vi "test Cluster Set and Get (enum).vi"(8 "error in (no error)":errorcluster, 11 "TestCase in":refnum<class "AIM ARINC 664 Scripting.lvclass">) -> (0 "error out":errorcluster, 3 "TestCase out":refnum<class "AIM ARINC 664 Scripting.lvclass">)   [LabVIEW 2020, in "AIM ARINC 664 Scripting.lvclass"]
uses:
  AIM ARINC 664 Scripting.lvclass
  C:/Program Files (x86)/National Instruments/LabVIEW 2020/vi.lib/addons/_JKI Toolkits/VI Tester/TestCase.llb/TestCase.lvclass
  Shared/loggingThreshold_types.ctl
  <vilib>/addons/_JKI Toolkits/VI Tester/TestCase.llb/TestCase.lvclass
  Scripting/AIM ARINC 664 Scripting.lvlib
panel:
  in  "in":T1={"Segmentation Threshold"=0.0, "Disk Space Percentage"=0.0, "Check Disk Space"=TRUE, "Segment File"=FALSE, "Segment Files By"=1} {"Segment Files By" items=["Time", "Size"]}
  out "out":T1 {"Segment Files By" items=["Time", "Size"]}
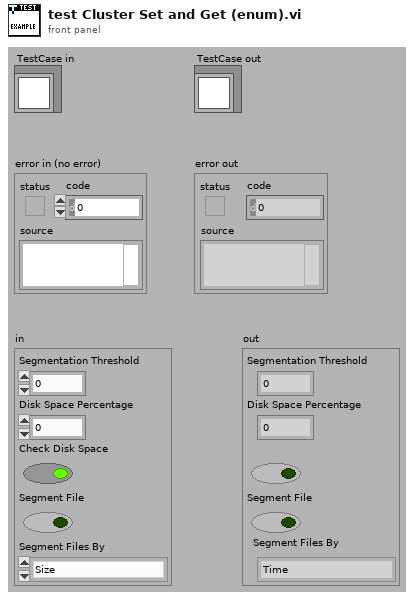
[diagram p1: front panel]
types:
  T1 = typedef "loggingThreshold_types.ctl" = cluster{"Segmentation Threshold":dbl, "Disk Space Percentage":dbl, "Check Disk Space":bool, "Segment File":bool, "Segment Files By":u16}
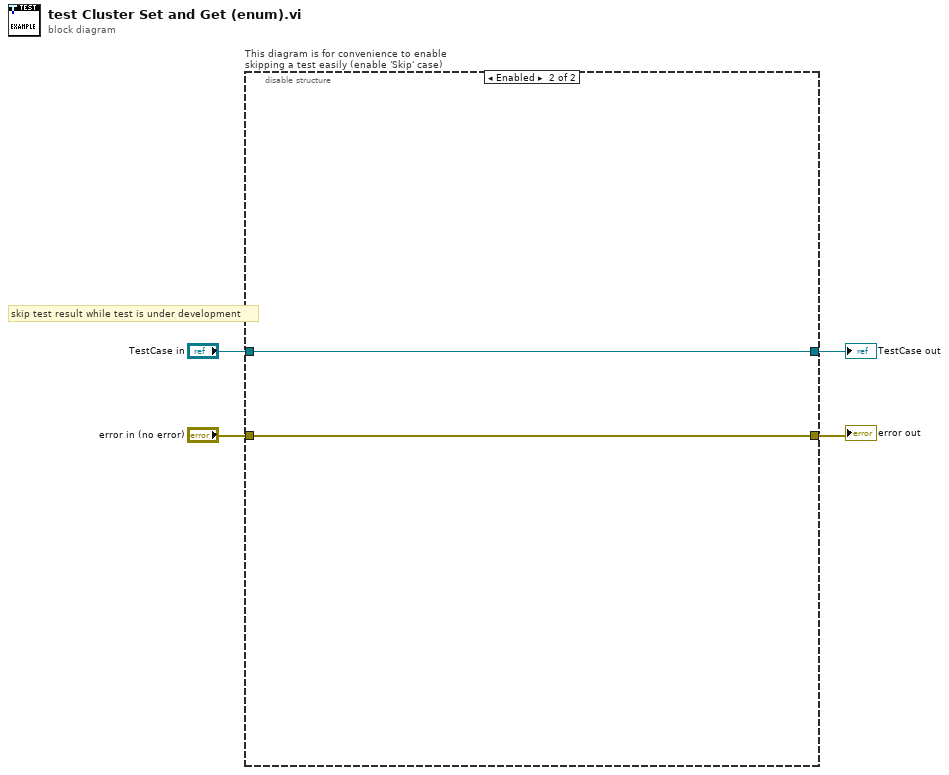
[diagram p0: block diagram]
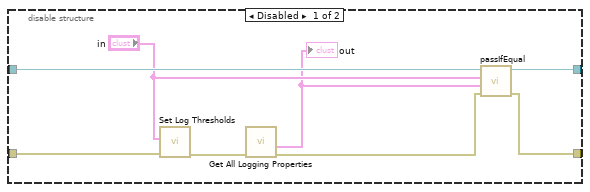
[diagram p2: hidden frame]
diagram:
  n1 = disable-structure "This diagram is for convenience to enable skipping a test easily (enable 'Skip' case)" shown="Enabled" {
    disable-tunnel: "TestCase in" -> [w10 w16]
    disable-tunnel: [w11 w14] -> w1
    disable-tunnel: [w12 w15] -> w3
    disable-tunnel: "error in (no error)" -> [w8 w13]
    frame Disabled {
      n2 = call "Set Log Thresholds.vi"("error in"=w8, "log thresholds"="in") -> ("error out"=w9:errorcluster)  [unwired: 8 in, 1 out]
      n3 = call "Get All Logging Properties.vi"("error in"=w9) -> ("error out"=w7:errorcluster, "log thresholds"=w5:T1)  [unwired: 7 in, 2 out]
      "out" <- w5
      n4 = call-dynamic "passIfEqual.vi"("error in (no error)"=w7, "y"=w5, "x"="in", "TestCase in"=w10) -> ("error out"=w12:errorcluster, "TestCase out"=w11:refnum<class "AIM ARINC 664 Scripting.lvclass">)  [unwired: 6 in]
    }
    frame Enabled {
      # "skip test result while test is under development"
      n5 = call <vilib>:"skip.vi"("error in (no error)"=w13, "TestCase in"=w16) -> ("error out"=w15:errorcluster, "TestCase out"=w14:refnum<class "AIM ARINC 664 Scripting.lvclass">)  [unwired: 8 in]
    }
  }
  "error out" <- w3
  "TestCase out" <- w1
